vi "Do.vi"(8 "error in (no error)":errorcluster, 10 "Actor in":refnum<class "Actor.lvclass">, 11 "Event Handler Msg":refnum<class "Event Handler Msg.lvclass">) -> (0 "error out":errorcluster, 2 "Actor out":refnum<class "Actor.lvclass">)   [LabVIEW 2026, in "TALOS.lvlib" / "Father of all uServices.lvlib" / "Event Handler Msg.lvclass"]
doc: "This VI delivers the message to the actor by calling the appropriate method(s) on the actor."
uses:
  Event Handler Msg.lvclass
  builds/Actor Framework PPL/Actor Framework.lvlibp/1abvi3w/vi.lib/ActorFramework/Actor/Actor.lvclass
  Event Handler Msg.lvclass/Event Handler Msg.ctl
  Father of all uServices/Father of all uServices.lvclass
  C:/LabVIEW Code/TALOS/builds/Actor Framework PPL/Actor Framework.lvlibp/1abvi3w/vi.lib/ActorFramework/Actor/Actor.lvclass
  57987545-233e-47b8-8de9-fafa71867b20.vi
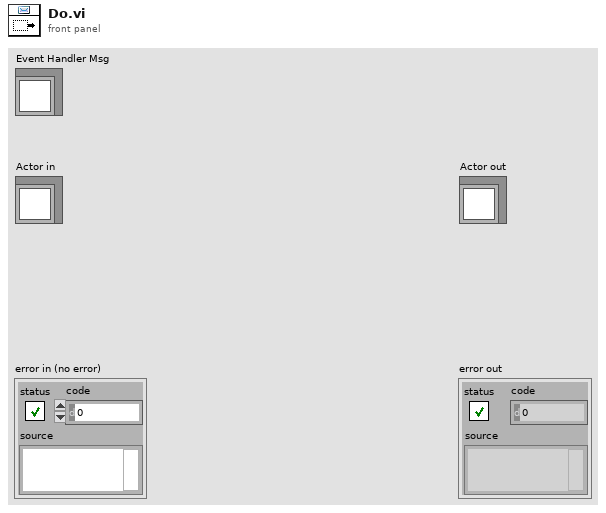
[diagram p1: front panel]
types:
  T1 = typedef "TALOS.lvlib/Father of all uServices.lvlib/Father of all uServices.lvclass/Event Handler Items.ctl" = enum16{"Button Pressed", "Message", "Ready to launch?", "Safe Mode", "Start RUN", "Stop RUN"}
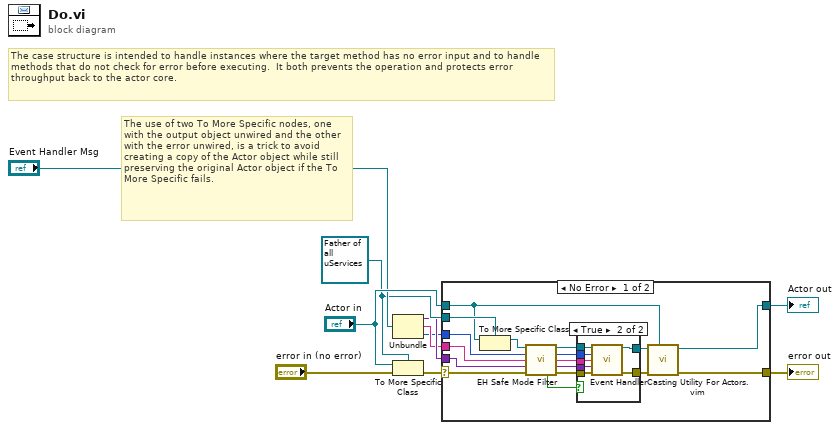
[diagram p0: block diagram]
diagram:
  w5 = refnum<class "Father of all uServices.lvclass"> refnum ("Actor in")
  # "The use of two To More Specific nodes, one with the output object unwired and the other with the error unwired, is a trick to avoid creating a copy of the Actor object while still preserving the original Actor object if the To More Specific fails."
  # "The case structure is intended to handle instances where the target method has no error input and to handle methods that do not check for error before executing.  It both prevents the operation and protects error throughput back to the actor core."
  n1 = Unbundle("Event Handler Msg") -> (w3:variant, w2:string, w1:T1)
  n2 = To More Specific Class(target class=w5, reference="Actor in", error in="error in (no error)") -> (error out=w4:errorcluster)  [unwired: 1 out]
  n3 = case shown="No Error" w4 {
    selector: w4 -> [w17 w38]
    tunnel: [w24 w38] -> w10
    tunnel: [w25 w37] -> w9
    tunnel: "Actor in" -> [w11 w37]
    tunnel: w5 -> [w27 _]
    tunnel: w3 -> [w18 _]
    tunnel: w2 -> [w19 _]
    tunnel: w1 -> [w20 _]
    frame No Error {
      n4 = To More Specific Class(target class=w27, reference=w11) -> (specific class reference=w22:refnum<class "Father of all uServices.lvclass">)  [unwired: 1 in, 1 out]
      n5 = call-dynamic "EH Safe Mode Filter.vi"("Father of all uServices in"=w22, "Event type"=w20, "Item Name"=w19, "Data"=w18, "error in (no error)"=w17) -> ("Father of all uServices out"=w21:refnum<class "Father of all uServices.lvclass">, "Event type out"=w13:T1, "Item Name out"=w14:string, "Data out"=w15:variant, "Execute"=w12:bool, "error out"=w16:errorcluster)  [unwired: 5 in]
      n6 = case shown="True" w12 {
        tunnel: [w29 w36] -> w26
        tunnel: [w28 w35] -> w23
        tunnel: w21 -> [w29 w34]
        tunnel: w16 -> [w28 w33]
        tunnel: w15 -> [_ w32]
        tunnel: w14 -> [_ w31]
        tunnel: w13 -> [_ w30]
        frame False {
        }
        frame True {
          n7 = call-dynamic "Event Handler.vi"("uService Template in"=w34, "Event type"=w30, "Item Name"=w31, "Data"=w32, "error in (no error)"=w33) -> ("uService Template out"=w36:refnum<class "Father of all uServices.lvclass">, "error out"=w35:errorcluster)  [unwired: 9 in]
        }
      }
      n8 = call "Casting Utility For Actors.vim"("type"=w11, "error in (no error)"=w23, "Actor in"=w26) -> ("error out"=w24:errorcluster, "Actor out"=w25:refnum<class "Actor.lvclass">)  [unwired: 7 in]
    }
    frame Error {
      # "If type check fails, pass the original object out again."
    }
  }
  "error out" <- w10
  "Actor out" <- w9
